vi "Error Handler.vi"(8 "error in (no error)":errorcluster, 10 "States In":string[](array[string]), 11 "Message":string) -> (0 "error out":errorcluster, 3 "States Out":string[](array[string]))   [LabVIEW 2018]
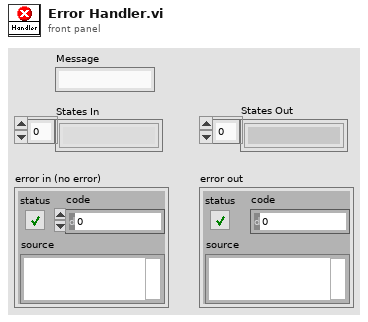
[diagram p1: front panel]
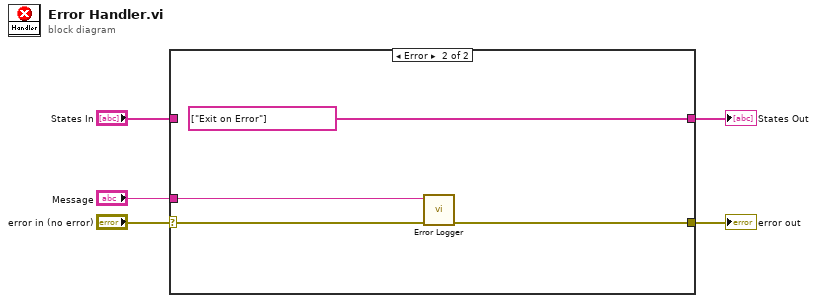
[diagram p0: block diagram]
diagram:
  n1 = case shown="Error" "error in (no error)" {
    selector: "error in (no error)" -> [w7 w9]
    tunnel: [w7 w10] -> w3
    tunnel: "States In" -> [w6 _]
    tunnel: [w6 string[] ["Exit on Error"]] -> w5
    tunnel: "Message" -> [_ w8]
    frame No Error {
    }
    frame Error {
      n2 = call "Error Logger.vi"("error in (no error)"=w9, "Message"=w8) -> ("error out"=w10:errorcluster)  [unwired: 9 in]
    }
  }
  "States Out" <- w5
  "error out" <- w3
